vi "Apollo_add_test_result.vi"(9 "Test stream":string) -> ()   [LabVIEW 2010]
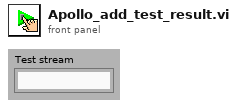
[diagram p1: front panel]
types:
  T1 = enum16{"open", "replace", "create", "open or create", "replace or create", "replace or create with confirmation"}
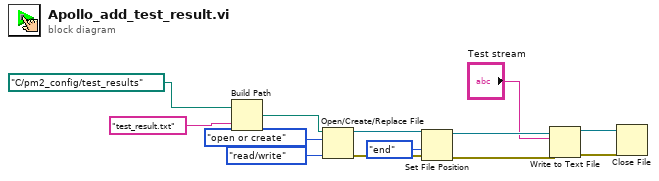
[diagram p0: block diagram]
diagram:
  n1 = Build Path(base path=path "C:/pm2_config/test_results" ("file path (use dialog)"), name or relative path="test_result.txt") -> (appended path=w13:path)
  n2 = Open/Create/Replace File(file path (use dialog)=w13, operation (0:open)=T1."open or create", access (0:read/write)=enum16{"read/write", "read-only", "write-only"}."read/write") -> (refnum out=w4:refnum<file>, error out=w6:errorcluster)  [unwired: 3 in, 1 out]
  n3 = Set File Position(refnum=w4, from (0:start)=enum16{"start", "end", "current"}."end", error in=w6) -> (refnum out=w3:refnum<file>, error out=w5:errorcluster)  [unwired: 1 in]
  n4 = Write to Text File(file (use dialog)=w3, text="Test stream", error in=w5) -> (refnum out=w10:refnum<file>, error out=w11:errorcluster)  [unwired: 1 in, 1 out]
  n5 = Close File(refnum=w10, error in=w11) -> ()  [unwired: 2 out]
